vi "xijk_load_vendor_removal_lines.vi"(11 "table in":string[][](array[string])) -> (3 "table out":string[][](array[string]))   [LabVIEW 2010]
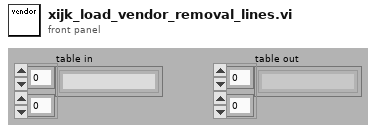
[diagram p1: front panel]
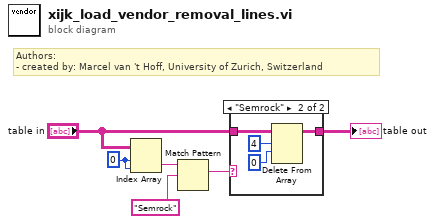
[diagram p0: block diagram]
diagram:
  w4 = 0 ("index (row)")
  # "Authors: \n- created by: Marcel van 't Hoff, University of Zurich, Switzerland"
  n1 = Index Array(array="table in", index (row)=w4, index (col)=w4) -> (element=w2:string)
  n2 = Match Pattern(string=w2, regular expression="Semrock") -> (match substring=w1:string)  [unwired: 4 out]
  n3 = case shown="\"Semrock\"" w1 {
    tunnel: "table in" -> [w7 w10]
    tunnel: [w7 w8] -> w6
    frame Default {
    }
    frame "Semrock" {
      n4 = Delete From Array(array=w10, length=4, index (row)=0 ("indice (ligne)")) -> (array with subset deleted=w8:string[][])  [unwired: 1 in, 1 out]
    }
  }
  "table out" <- w6
